vi "GenerateCode.vi"(1 "Terms":T1[](array[typedef]), 3 "Diagram":refnum<vi>, 5 "XRef":refnum<vi>, 6 "State In":T4={"Input Type"=variant(path path ""), "Terminals"=[]}) -> (0 "Generated Code?":bool, 2 "State Out":T4={"Input Type"=variant(path path ""), "Terminals"=[]}, 4 "Reply":string[](array[string]))   [LabVIEW 2015, in "Await.xnode"]
doc: "This ability VI is called when it is time to define the execution behavior of your XNode via LabVIEW's scripting API. This VI is only called when you have previously informed LabVIEW that you need to script through a GenerateCode reply. Diagram is a reference to a diagram of a temporary VI. This diagram contains exactly one front panel terminal for each terminal of your XNode. Terms is an array of pairs of Term IDs and terminal references. LabVIEW will copy code scripted into this diagram into your XNode and connect everything to the correct terminals. The front panel terminals that are on this diagram are special in that they can only be on the top level diagram.\n \n Generate Code? is used to tell LabVIEW whether or not you want to copy the scripted diagram over. If there is an error and you wish not to commit the changes, then the old XNode behavior will be left unchanged. If you set Generate Code? to false, then this VI will be called again next time type propagation is run. Otherwise, it will not be called until you indicate that it should be through the reply on another ability VI.\n \n Because the diagram you are scripting into is separate from the VI containing the XNode instance, type propagation and the data manager will run on the temporary VI after each scripting call.\n \n You should not use the Copy scripting method to move code into the temporary VI. This will adversely affect the user's clipboard. You should use the Move scripting method instead.\n\nDefault behavior: None.\n\nThis ability does not provide UI and OS messages are not handled.\n\nSee also: ModifyCode"
uses:
  Await.xnode
  State.ctl
  <vilib>/XNodeSupport/XNodeTermIDPair.ctl
  <vilib>/XNodeSupport/XNodeTermRef.ctl
  <vilib>/XNodeSupport/XNodeString.ctl
  <vilib>/Erdos Miller/LV-Scripting/LV-Scripting.lvlib
  <vilib>/Erdos Miller/LV-VI/LV-VI.lvlib
  <vilib>/XNodeSupport/NI_XNodeSupport.lvlib
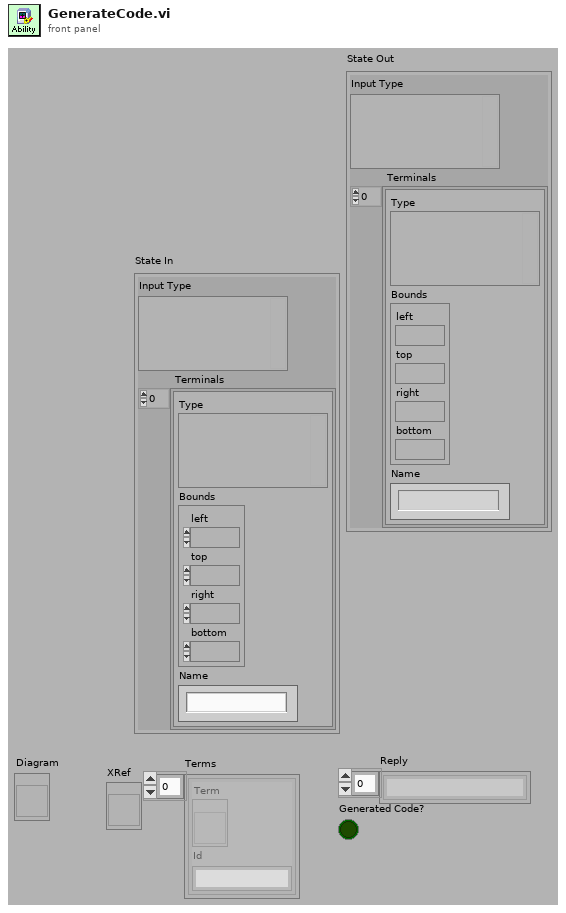
[diagram p1: front panel]
types:
  T1 = typedef "NI_XNodeSupport.lvlib/XNodeTermIDPair.ctl" = cluster{"Term":T2, "Id":T3}
  T2 = typedef "NI_XNodeSupport.lvlib/XNodeTermRef.ctl" = refnum<vi>
  T3 = typedef "NI_XNodeSupport.lvlib/XNodeString.ctl" = string
  T4 = typedef "Await.xnode/State.ctl" = cluster{"Input Type":variant, "Terminals":cluster{"Type":variant, "Bounds":cluster{"left":i16, "top":i16, "right":i16, "bottom":i16}, "Name":string}[]}
  T5 = cluster{"Type":variant, "Bounds":cluster{"left":i16, "top":i16, "right":i16, "bottom":i16}, "Name":string}[]
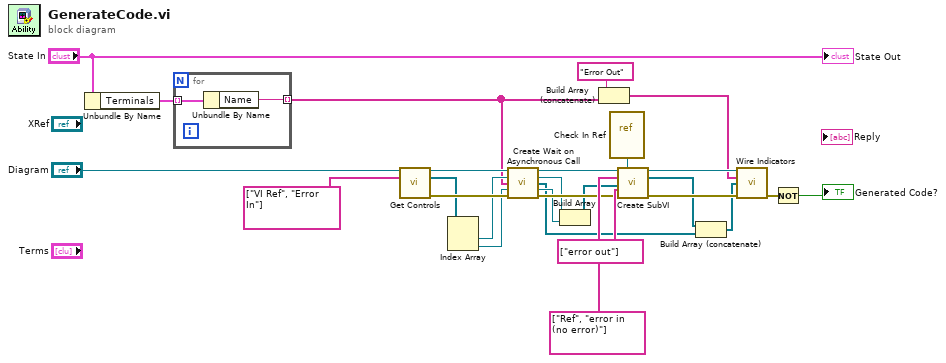
[diagram p0: block diagram]
diagram:
  n1 = Unbundle By Name("State In") -> ("Terminals"=w26:T5)
  n2 = for {
    tunnel: w26 -> [w29] mode=indexing
    tunnel: [w28] -> w8 mode=indexing
    n3 = Unbundle By Name(w29) -> ("Name"=w28:string)
  }
  n4 = call <vilib>:"Get Controls.vi"("Diagram in"="Diagram", "Control Names"=string[] ["VI Ref", "Error In"] ("element")) -> ("Diagram out"=w23:refnum<vi>, "Control Terminals"=w21:refnum<vi>[], "error out"=w22:errorcluster)  [unwired: 11 in]
  n5 = Index Array(array=w21) -> (element #1=w20:refnum<vi>, element #2=w19:refnum<vi>)  [unwired: 2 in]
  n6 = call <vilib>:"Create Wait on Asynchronous Call.vi"("Diagram in"=w23, "reference"=w20, "Output Names"=w8, "error in"=w19, "error in (no error)"=w22) -> ("Diagram out"=w18:refnum<vi>, "reference out"=w13:refnum<vi>, "Outputs"=w4:refnum<vi>[], 10:"error out"=w12:refnum<vi>, 15:"error out"=w14:errorcluster)  [unwired: 6 in]
  n7 = Build Array(w13, w12) -> (w11:refnum<vi>[])
  n8 = Build Array (concatenate)("Error Out", w8) -> (w6:string[])
  n9 = vi-ref <vilib>:"Check In Ref.vi"() -> (w17:refnum<vi>)
  n10 = call <vilib>:"Create SubVI.vi"("Diagram in"=w18, "VI Reference"=w17, "Input Names"=string[] ["Ref", "error in (no error)"], "Inputs"=w11, "Output Names"=string[] ["error out"], "error in (no error)"=w14) -> ("Diagram out"=w10:refnum<vi>, "Outputs"=w3:refnum<vi>[], "error out"=w9:errorcluster)  [unwired: 7 in]
  n11 = Build Array (concatenate)(w3, w4) -> (w2:refnum<vi>[])
  n12 = call <vilib>:"Wire Indicators.vi"("Diagram in"=w10, "Indicator Names"=w6, "Outputs"=w2, "error in (no error)"=w9) -> ("error out"=w7:errorcluster)  [unwired: 10 in, 1 out]
  n13 = Not(x=w7) -> (.not. x?=→"Generated Code?":bool)
  "State Out" <- "State In"
